vi "TrazarRuta (Sub VI).vi"(0 "LAT INI":string="-2.907134", 1 "LNG INI":string="-79.018658", 2 "LAT END":string="-2.897034", 3 "LNG END":string="-79.007658") -> (5 "URL":string)   [LabVIEW 2012]
uses:
  <vilib>/Utility/NIReport.llb/NI_report.lvclass
panel:
  in  "HTML Save Path":path caption="HTML Save Path (if empty, uses example.html in temp directory)"
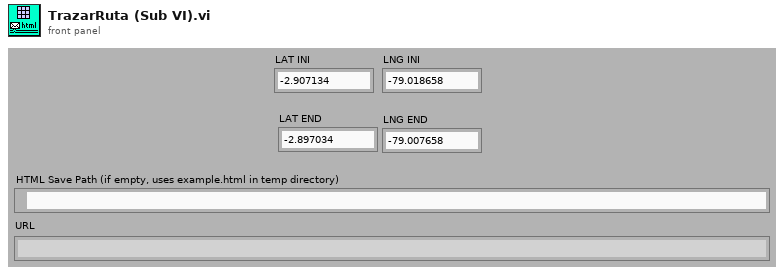
[diagram p1: front panel]
types:
  T1 = enum16{"Standard Report", "HTML", "Word", "Excel"}
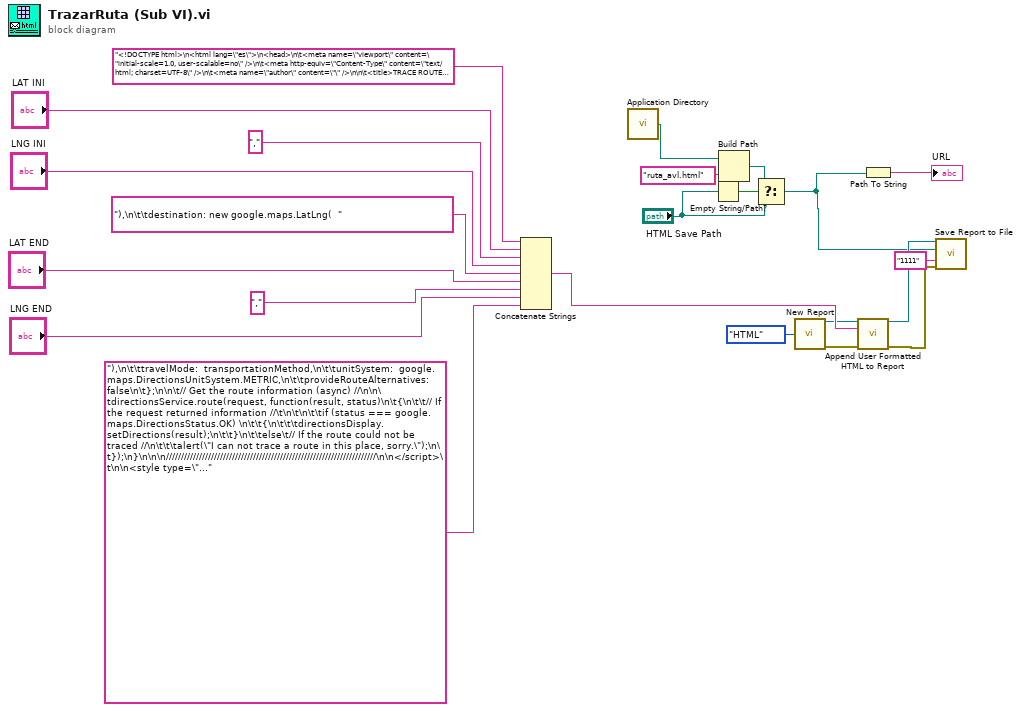
[diagram p0: block diagram]
diagram:
  n1 = Concatenate Strings("<!DOCTYPE html>\n<html lang=\"es\">\n<head>\n\t<meta name=\"viewport\" content=\"initial-scale=1.0, user-scalable=no\" />\n\t<meta http-equiv=\"Content-Type\" content=\"text/html; charset=UTF-8\" />\n\t<meta name=\"author\" content=\"\" />\n\n\t<title>TRACE ROUTE</title>\n\t\t\n\t<script type=\"text/javascript\" src=\"http://maps.google.com/maps/api/js?sensor=false&language=es\"></script>\n\t  \n<script type='text/javascript'>\n\n/******************************************************************\n\n   ******************************************************************/\n\n//////////////////////////////////////////////////////////////////////\n\n// Current location data //\n\nvar currentLocation = {\n\tlatitude:         -2.900005,\n\tlongitude:        -78.983335,\n\treal:             false,\n\taltitude:         null,\n\taccuracy:         null,\n\taltitudeAccuracy: null,\n\theading:          null,\n\tspeed:            null\n};\n\n// Reference to the whole map //\n\nvar map = null;\t\n\n\t\n\n// References to the Google services to display routes and //\n// get directions                                          //\n\nvar directionsService = new google.maps.DirectionsService();\nvar directionsDisplay = new google.maps.DirectionsRenderer();\n\n/**\n * Code block executed as soon as the page is loaded.\n */  \n\nwindow.onload = function() \n{\n\t// Setup the map infraestructure //\n\n\tsetupMap();\n\t\n\t// Associate the Go! button with its action handler //\t\n\n\t\n\t// Associate the change of transportation method with its action handler //\t\n\n\tdocument.getElementById('transportation_method').onchange = function(event) {\n\t\ttraceRoute();\n\t};\t\n}\n\n//////////////////////////////////////////////////////////////////////\n\n/**\n * Setup the map in its initial stage: gets the geolocation information (if available),\n * invokes the map creation and locates the user current location marker\n */\n\nfunction setupMap()\n{\n\t// Test if the geolocation feature is available //\n\n\t//if (navigator.geolocation) \n\t\n\t\n\t\tmap = createMap(currentLocation.latitude, currentLocation.longitude);\t\n\t\n\t//smul\taddYou();\t\n\t\n\t\n}\n\n/**\n * Creates a map using the Google Maps API and \n * centered in the specified location\n */\n\nfunction createMap(latitude, longitude)\n{\n\t// Create the map //\n\n\tvar mapDiv = document.getElementById('map');\n\t\n\tvar latlng = new google.maps.LatLng(latitude, longitude);\n\t\n\tvar options = {\n\t\tcenter: latlng,\n\t\tzoom: 15,\n\t\t\n\t\tmapTypeId: google.maps.MapTypeId.TERRAIN\n\t};\n\t\n\tmap = new google.maps.Map(mapDiv, options);\n\t\n\t// Relate the map and the directions DIV with // \n\t// the service provider reference             //\t\n\t\n\tdirectionsDisplay.setMap(map);\n\t\n\tdirectionsDisplay.setPanel(document.getElementById(\"map_directions\"));\n\t\n\t// Relates the click event over the map with the //\n\t// location of the destinations marker           //\t\n\t\n traceRoute();\n\n\treturn map;\n}\n\n//////////////////////////////////////////////////////////////////////\n\n/**\n * Adds a marker to the map with the specified information\n */\n\n\n\nfunction addMarker(map, latitude, longitude, tooltip, message, icon)\n{\n\t// Basic marker information //\n\n\tvar marker = new google.maps.Marker({\n\t\tposition: new google.maps.LatLng(latitude, longitude),\n\t\tmap:      map,\n\t\ttitle:    tooltip\n\t});\n\t\n\t// Set a different icon if specified //\t\n\t\n\treturn marker;\n}\n\n\n\n//////////////////////////////////////////////////////////////////////\n\n/**\n * Create the marker for the destination in the specified location\n */\n\nfunction addDestination(latitude, longitude)\n{\n\t// If exists previously, remove it first //\n\n\tif(she != null)\n\t\tshe.setMap(null);\n\n\tshe = addMarker(map, latitude, longitude, 'Destination', null, 'img/destination.png');\n\t\n\t// When destination is provided, trace a route between \"you\" and \"destination\" //\t\n\t\n\ttraceRoute();\n}\n\n//////////////////////////////////////////////////////////////////////\n\n/**\n * Get the route and direction information to get from \"you\"\n * to the destination point using the Google's service\n */\n\nfunction traceRoute()\n{\n\t// Verify that destination is really available //\n\t\n//\tif(she == null)\n//\t\treturn false;\n\n\t// Define the transportation method //\n\t\n\tvar transportationMethod = google.maps.DirectionsTravelMode.WALKING; \t\n\t\n\tif (document.getElementById('transportation_method').value == \"DRIVING\")\n\t\ttransportationMethod = google.maps.DirectionsTravelMode.DRIVING;\n\n\tif (document.getElementById('transportation_method').value == \"WALKING\")\n\t\ttransportationMethod = google.maps.DirectionsTravelMode.WALKING;\n\n\t// Set the service's request information //\n\n\tvar request = {\n\t\torigin:      new google.maps.LatLng( " ("Table Headers"), "LAT INI", "," ("Table Headers"), "LNG INI", "),\n\t\tdestination: new google.maps.LatLng(  " ("Table Headers"), "LAT END", "," ("Table Headers"), "LNG END", "),\n\t\ttravelMode:  transportationMethod,\n\t\tunitSystem:  google.maps.DirectionsUnitSystem.METRIC,\n\t\tprovideRouteAlternatives: false\n\t};\n\n\t// Get the route information (async) //\n\n\tdirectionsService.route(request, function(result, status)\n\t{\n\t\t// If the request returned information //\t\n\t\n\t\tif (status === google.maps.DirectionsStatus.OK) \n\t\t{\n\t\t\tdirectionsDisplay.setDirections(result);\n\t\t}\n\t\telse\t// If the route could not be traced //\n\t\t\talert(\"I can not trace a route in this place, sorry.\");\n\t});\n}\n\n\n//////////////////////////////////////////////////////////////////////\n\n</script>\t\n\n<style type=\"text/css\">\n\na\n{\n\tcolor: #809F00;\n\ttext-decoration: none;\n}\n\n#page\n{\n\twidth: 1000px;\n\theight: 490px;\n\tmargin: 1px;\n\tfont-family: verdana,helvetica,arial,sans-serif;\n}\n\n#head\n{\n\tpadding-bottom: 1px;\n\tmargin-bottom: 1px;\n}\n\n\n\n#map\n{\n\twidth: 710px;\n\theight: 490px;\n\tfloat: left;\n\toverflow: auto;\n}\n\n#map_directions\n{\n\twidth: 250px;\n\theight: 450px;\n\tfloat: right;\n\tfont-size: 0.7em;\n\toverflow: auto;\n\n}\n\n#transportation_bar\n{\n\tpadding-bottom: 8px;\n\ttext-align: right;\n}\n\n#transportation_bar #title\n{\n\tfont-size: 0.7em;\n\tfont-weight: bold;\n\tpadding: 5px 15px 0px 20px;\n}\n\n#transportation_bar select\n{\n\theight: 25px;\n\tborder-style: ridge;\n\tfont-size: 17px;\n}\n\n#foot\n{\n\n   \tfloat: right;\n\toverflow: auto;\n\ttext-align: right;\n\tfont-size: 0.8em;\n\tpadding-top: 5px;\n\tmargin-top: 5px;\n}\n\n#foot #left\n{\n\tfloat: left;\n}\n\n#foot #right\n{\n\tfloat: right;\n}\n\n#foot #license\n{\n\tborder: 0;\n\tvertical-align: middle;  \n}\n\n.bubble\n{\n\twidth: 500px;\n\tfont-size: 0.8em;\n}\n\n</style>\n</head>\n\n<body>\n\n<body bgcolor=\"#CCCCCC\">\n\n<div id='page'>\n\t<div id='head'>\n\t\n\t</div>\n\n\t<div id=\"transportation_bar\">\n\t\t<span id=\"title\">Transportation method</span>\n\t\t<select id=\"transportation_method\">\n\t\t\t<option value=\"DRIVING\">Driving</option>\n\t\t\t<option value=\"WALKING\">Walking</option>\n\t\t</select>\t\t\n\t</div>\n\n\t<div id=\"middle\">\n\t\t<div id='map'>\n\t\t</div>\n\t\n\t\t<div id='map_directions'>\n\t\t\tThere are no directions available!\n\t\t</div>\n\t</div>\n\n\n\n\t<div id='foot'>\n\t\t<div id='left'>\n\t\t\n\t\t</div>\n\t\t<div id='right'>\n\t\t\tDeveloped by <a href='http://sandrouday.com/' target='_blank'>SANDRO UDAY LUPERCIO</a>.\n\t\t</div>\n\t</div>\n</div>\n\t\n</body>\t\n</html>\n" ("Table Headers")) -> (w23:string)
  n2 = call <vilib>:"Application Directory.vi"() -> ("Application Directory"=w1:path)
  n3 = Empty String/Path?(string/path="HTML Save Path") -> (empty?=w9:bool)
  n4 = Build Path(base path=w1, name or relative path="ruta_avl.html") -> (appended path=w8:path)
  n5 = Select(t=w8, s=w9, f="HTML Save Path") -> (s? t:f=w3:path)
  n6 = call <vilib>:"New Report.vi"("report type"=T1."HTML") -> ("report out"=w12:refnum<class "NI_report.lvclass">, "error out"=w11:errorcluster)  [unwired: 5 in, 8 out]
  n7 = call-dynamic "Append User Formatted HTML to Report.vi"("report in"=w12, "HTML text"=w23, "error in (no error)"=w11) -> ("report out"=w6:refnum<class "NI_report.lvclass">, "error out"=w5:errorcluster)  [unwired: 11 out]
  n8 = Path To String(path=w3) -> (string=→"URL":string)
  n9 = call-dynamic "Save Report to File.vi"("report in"=w6, "report file path"=w3, "password (\"\")"="1111" ("password (\"\")"), "error in (no error)"=w5) -> ()  [unwired: 10 in, 2 out]
